vi "Configure Modulation Low Level (PM Deviation).vi"(8 "error in":errorcluster, 10 "Peak Deviation (180 degrees)":i32=180 min=0 max=360, 11 "VISA resource name":refnum<visa-resource-name>) -> (0 "error out":errorcluster, 3 "VISA resource name out":refnum<visa-resource-name>)   [LabVIEW 2017, in "Keithley 3390.lvlib"]
doc: "Sets the phase deviation of the phase modulation technique. The phase deviation represents the peak variation of the modulation output based on theat of the carrier waveform."
uses:
  Keithley 3390.lvlib
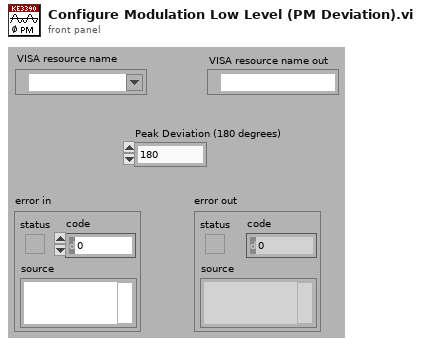
[diagram p1: front panel]
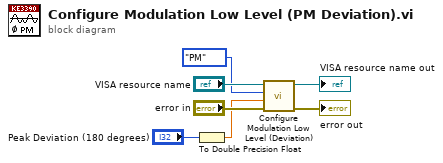
[diagram p0: block diagram]
diagram:
  n1 = To Double Precision Float(number="Peak Deviation (180 degrees)") -> (double precision float=w2:dbl)
  n2 = call "Configure Modulation Low Level (Deviation).vi"("error in (no error)"="error in", "Deviation"=w2, "Modulation (FM)"=enum16{"FM", "PM", "PWM"}."PM" ("Modulation (0: FM)"), "VISA resource name"="VISA resource name") -> ("error out"=→"error out":errorcluster, "VISA resource name out"=→"VISA resource name out":refnum<visa-resource-name>)  [unwired: 6 in]
